vi "Build Numeric Vars.vi"   [LabVIEW 2019]
uses:
  <vilib>/numeric/LVNumericRepresentation.ctl
types:
  T1 = typedef "LVNumericRepresentation.ctl" = enum32{"Extended Precision", "Double Precision", "Single Precision", "Long", "Word", "Byte", "Unsigned Long", "Unsigned Word", "Unsigned Byte", "Complex Extended", "Complex Double", "Complex Single", "Quad", "Unsigned Quad", "Fixed-Point"}
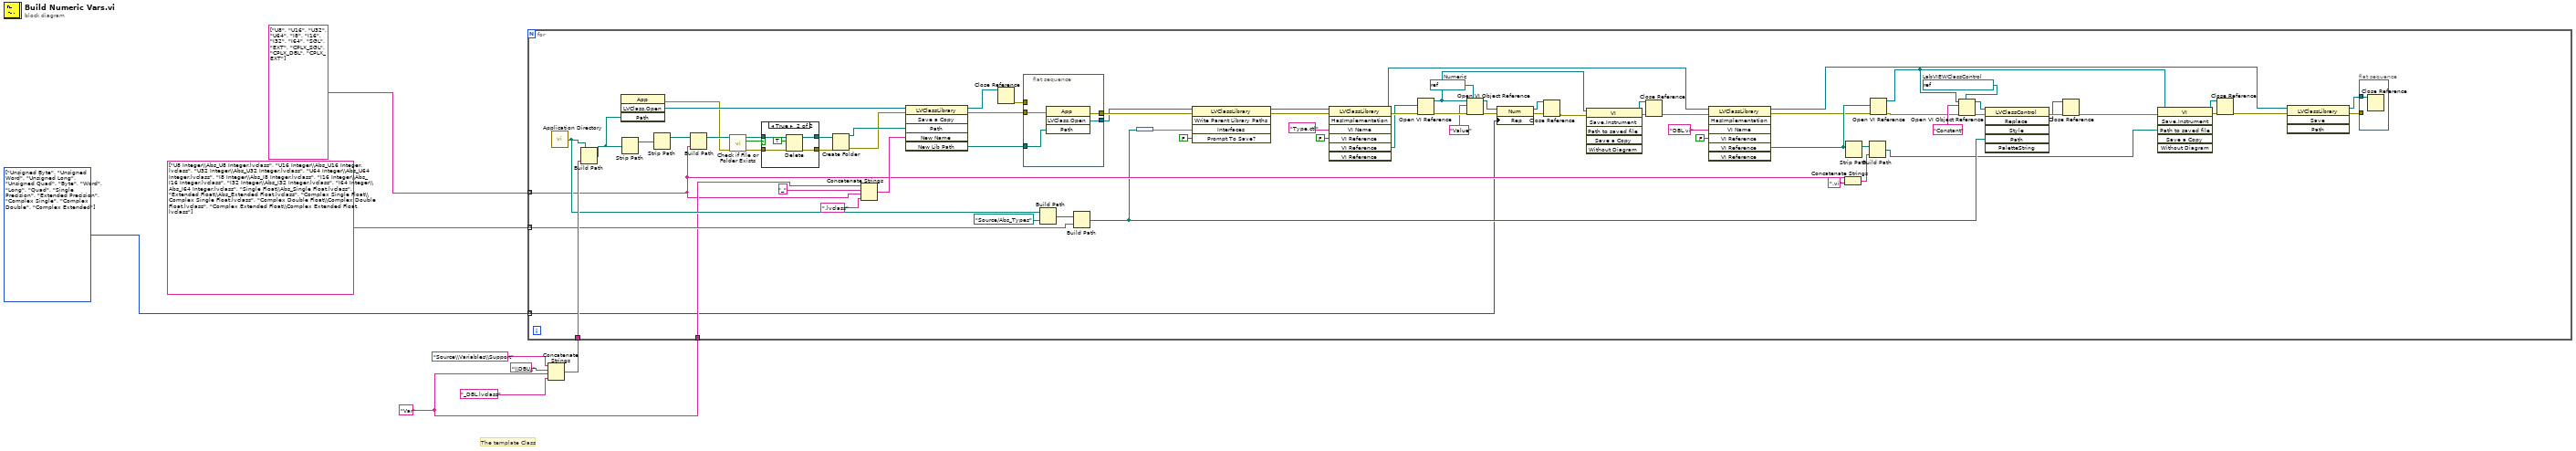
[diagram p0: block diagram]
diagram:
  w3 = T1[] [enum."Unsigned Byte", enum."Unsigned Word", enum."Unsigned Long", enum."Unsigned Quad", enum."Byte", enum."Word", enum."Long", enum."Quad", enum."Single Precision", enum."Extended Precision", enum."Complex Single", enum."Complex Double", enum."Complex Extended"] items=["Extended Precision", "Double Precision", "Single Precision", "Long", "Word", "Byte", "Unsigned Long", "Unsigned Word", "Unsigned Byte", "Complex Extended", "Complex Double", "Complex Single", "Quad", "Unsigned Quad", "Fixed-Point"] ("Representation")
  w8 = "Var" ("Comparison Name")
  # "The template Class"
  n1 = Concatenate Strings("Source\\Variables\\Support", "\\DBL\\", w8, "_DBL.lvclass") -> (w7:string)
  n2 = for {
    tunnel: string[] ["U8", "U16", "U32", "U64", "I8", "I16", "I32", "I64", "SGL", "EXT", "CPLX_SGL", "CPLX_DBL", "CPLX_EXT"] -> [w37] mode=indexing
    tunnel: w7 -> [w64]
    tunnel: string[] ["U8 Integer\\Abs_U8 Integer.lvclass", "U16 Integer\\Abs_U16 Integer.lvclass", "U32 Integer\\Abs_U32 Integer.lvclass", "U64 Integer\\Abs_U64 Integer.lvclass", "I8 Integer\\Abs_I8 Integer.lvclass", "I16 Integer\\Abs_I16 Integer.lvclass", "I32 Integer\\Abs_I32 Integer.lvclass", "I64 Integer\\Abs_I64 Integer.lvclass", "Single Float\\Abs_Single Float.lvclass", "Extended Float\\Abs_Extended Float.lvclass", "Complex Single Float\\Complex Single Float.lvclass", "Complex Double Float\\Complex Double Float.lvclass", "Complex Extended Float\\Complex Extended Float.lvclass"] -> [w58] mode=indexing
    tunnel: w3 -> [w20] mode=indexing
    tunnel: w8 -> [w48]
    w28 = refnum<vi> refnum  # Numeric
    w42 = refnum<vi> refnum  # LabVIEWClassControl
    n3 = call <vilib>:"Application Directory.vi"() -> ("Application Directory"=w53:path)
    n4 = Build Path(base path=w53, name or relative path=w64) -> (appended path=w65:path)
    n5 = invoke class="App" method="LVClass.Open"("Path"=w65) -> (error out=w70:errorcluster, "LVClass.Open"=w83:refnum<vi>)  [unwired: 3 in, 2 out]
    n6 = Strip Path(path=w65) -> (stripped path=w81:path)  [unwired: 1 out]
    n7 = Strip Path(path=w81) -> (stripped path=w80:path)  [unwired: 1 out]
    n8 = Build Path(base path=w80, name or relative path=w37) -> (appended path=w76:path)
    n9 = call <vilib>:"Check if File or Folder Exists.vi"("error in (no error)"=w70, "path"=w76) -> ("error out"=w69:errorcluster, "file or folder exists?"=w78:bool, "dup path"=w79:path)  [unwired: 7 in]
    n10 = case shown="True" w78 {
      tunnel: w79 -> [w90 w95]
      tunnel: [w90 w93] -> w77
      tunnel: w69 -> [w89 w92]
      tunnel: [w89 w91] -> w68
      frame False {
      }
      frame True {
        n11 = Delete(path (use dialog)=w95, entire hierarchy (F)=TRUE, error in=w92) -> (deleted path=w93:path, error out=w91:errorcluster)  [unwired: 2 in, 1 out]
      }
    }
    n12 = Create Folder(path (use dialog)=w77, error in=w68) -> (created path=w75:path, error out=w67:errorcluster)  [unwired: 1 in, 1 out]
    n13 = Concatenate Strings(w48, "_", w37, ".lvclass") -> (w63:string)
    n14 = invoke class="LVClassLibrary" method="Save a Copy"(reference=w83, error in=w67, "Path"=w75, "New Name"=w63) -> (reference out=w82:refnum<vi>, error out=w71:errorcluster, "New Lib Path"=w72:path)  [unwired: 2 in, 3 out]
    n15 = Close Reference(reference=w82) -> (error out=w66:errorcluster)  [unwired: 1 in]
    n16 = flat-sequence {
      tunnel: w72 -> [w87]
      tunnel: w71 -> [w88]
      tunnel: w66 -> [_]
      tunnel: [w85] -> w9
      tunnel: [w86] -> w52
      frame #0 {
        n17 = invoke class="App" method="LVClass.Open"(error in=w88, "Path"=w87) -> (error out=w86:errorcluster, "LVClass.Open"=w85:refnum<vi>)  [unwired: 2 in, 2 out]
      }
    }
    n18 = Build Path(base path=w53, name or relative path=path "Source/Abs_Types") -> (appended path=w59:path)
    n19 = Build Path(base path=w59, name or relative path=w58) -> (appended path=w35:path)
    n20 = node(w35) -> (w51:set{path})
    n21 = invoke class="LVClassLibrary" method="Write Parent Library Paths"(reference=w9, error in=w52, "Interfaces"=w51, "Prompt To Save?"=FALSE) -> (reference out=w30:refnum<vi>, error out=w31:errorcluster)  [unwired: 1 in, 3 out]
    n22 = invoke class="LVClassLibrary" method="HasImplementation"(reference=w30, error in=w31, "VI Name"="Type.ctl", "VI Reference"=FALSE ("Consider Parents?")) -> (reference out=w13:refnum<vi>, error out=w22:errorcluster, "VI Reference"=w15:path)  [unwired: 3 in, 4 out]
    n23 = Open VI Reference(vi path=w15, error in (no error)=w22) -> (vi reference=w16:refnum<vi>, error out=w29:errorcluster)  [unwired: 4 in]
    n24 = Open VI Object Reference(7:w28, 8:w29, 10:"Value" ("name/order"), 11:w16) -> (0:w27:errorcluster, 3:w26:refnum<vi>)
    n25 = property class="Num"(reference=w26, error in=w27, "Rep"=w20) -> (reference out=w25:refnum<vi>, error out=w24:errorcluster)
    n26 = Close Reference(reference=w25, error in (no error)=w24) -> (error out=w17:errorcluster)
    n27 = invoke class="VI" method="Save.Instrument"(reference=w16, error in=w17) -> (reference out=w19:refnum<vi>, error out=w18:errorcluster)  [unwired: 4 in, 4 out]
    n28 = Close Reference(reference=w19, error in (no error)=w18) -> (error out=w14:errorcluster)
    n29 = invoke class="LVClassLibrary" method="HasImplementation"(reference=w13, error in=w14, "VI Name"="DBL.vi", "VI Reference"=FALSE ("Consider Parents?")) -> (reference out=w11:refnum<vi>, error out=w12:errorcluster, "VI Reference"=w40:path)  [unwired: 3 in, 4 out]
    n30 = Concatenate Strings(w37, ".vi" ("string")) -> (w38:string)
    n31 = Strip Path(path=w40) -> (stripped path=w39:path)  [unwired: 1 out]
    n32 = Build Path(base path=w39, name or relative path=w38) -> (appended path=w10:path)
    n33 = Open VI Reference(vi path=w40, error in (no error)=w12) -> (vi reference=w34:refnum<vi>, error out=w21:errorcluster)  [unwired: 4 in]
    n34 = Open VI Object Reference(7:w42, 8:w21, 10:"Constant" ("name/order"), 11:w34) -> (0:w46:errorcluster, 3:w47:refnum<vi>)
    n35 = invoke class="LVClassControl" method="Replace"(reference=w47, error in=w46, "Path"=w35) -> (error out=w44:errorcluster, "Replace"=w43:refnum<vi>)  [unwired: 3 in, 4 out]
    n36 = Close Reference(reference=w43, error in (no error)=w44) -> (error out=w41:errorcluster)
    n37 = invoke class="VI" method="Save.Instrument"(reference=w34, error in=w41, "Path to saved file"=w10) -> (reference out=w49:refnum<vi>, error out=w50:errorcluster)  [unwired: 3 in, 4 out]
    n38 = Close Reference(reference=w49, error in (no error)=w50) -> (error out=w57:errorcluster)
    n39 = invoke class="LVClassLibrary" method="Save"(reference=w11, error in=w57) -> (reference out=w54:refnum<vi>, error out=w55:errorcluster)  [unwired: 2 in, 2 out]
    n40 = flat-sequence {
      tunnel: w54 -> [w84]
      tunnel: w55 -> [_]
      frame #0 {
        n41 = Close Reference(reference=w84) -> ()  [unwired: 1 in, 1 out]
      }
    }
  }
